vi "Get_WT_Speed.vi"(2 "Time (s)":dbl[](array[numeric]) format="%.4f", 3 "Av Sampling Rate":dbl, 4 "Opto Trace":dbl[](array[numeric]) format="%.2f") -> (0 "Time per Cycle":dbl[](array[numeric]), 1 "Start Cycle Time":dbl[](array[numeric]))   [LabVIEW 2021]
uses:
  <vilib>/Analysis/6fits.llb/Curve Fitting Criteria.ctl
  <vilib>/Analysis/baseanly.llb/Mean (DBL).vi
  <vilib>/Analysis/NI_AALBase.lvlib
  <vilib>/Analysis/NI_AALPro.lvlib
panel:
  out "Samples per cycle 1st":i32[](graph)
  out "Time (s) per cycle":dbl[](graph)
  out "Threshold value":dbl
  out "1/60 of cycle":i32
  out "Average samples per cycle":dbl format="%0.2f"
  out "No Of Cycles":i32
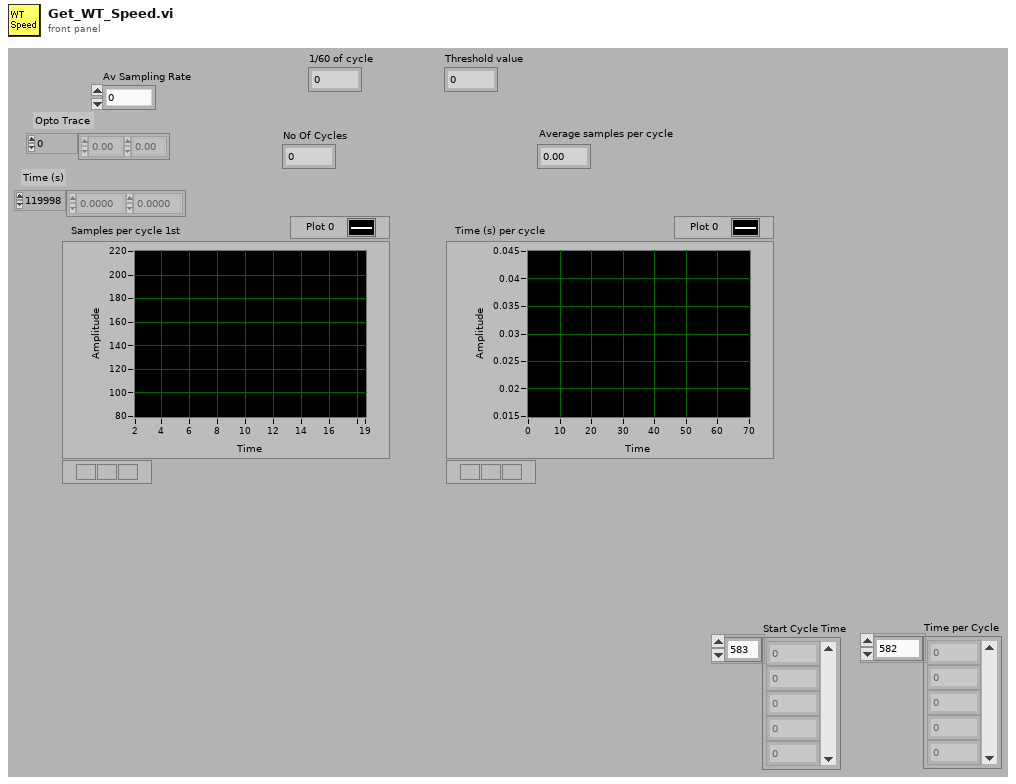
[diagram p1: front panel]
types:
  T1 = typedef "NI_AALPro.lvlib/Curve Fitting Criteria.ctl" = u16
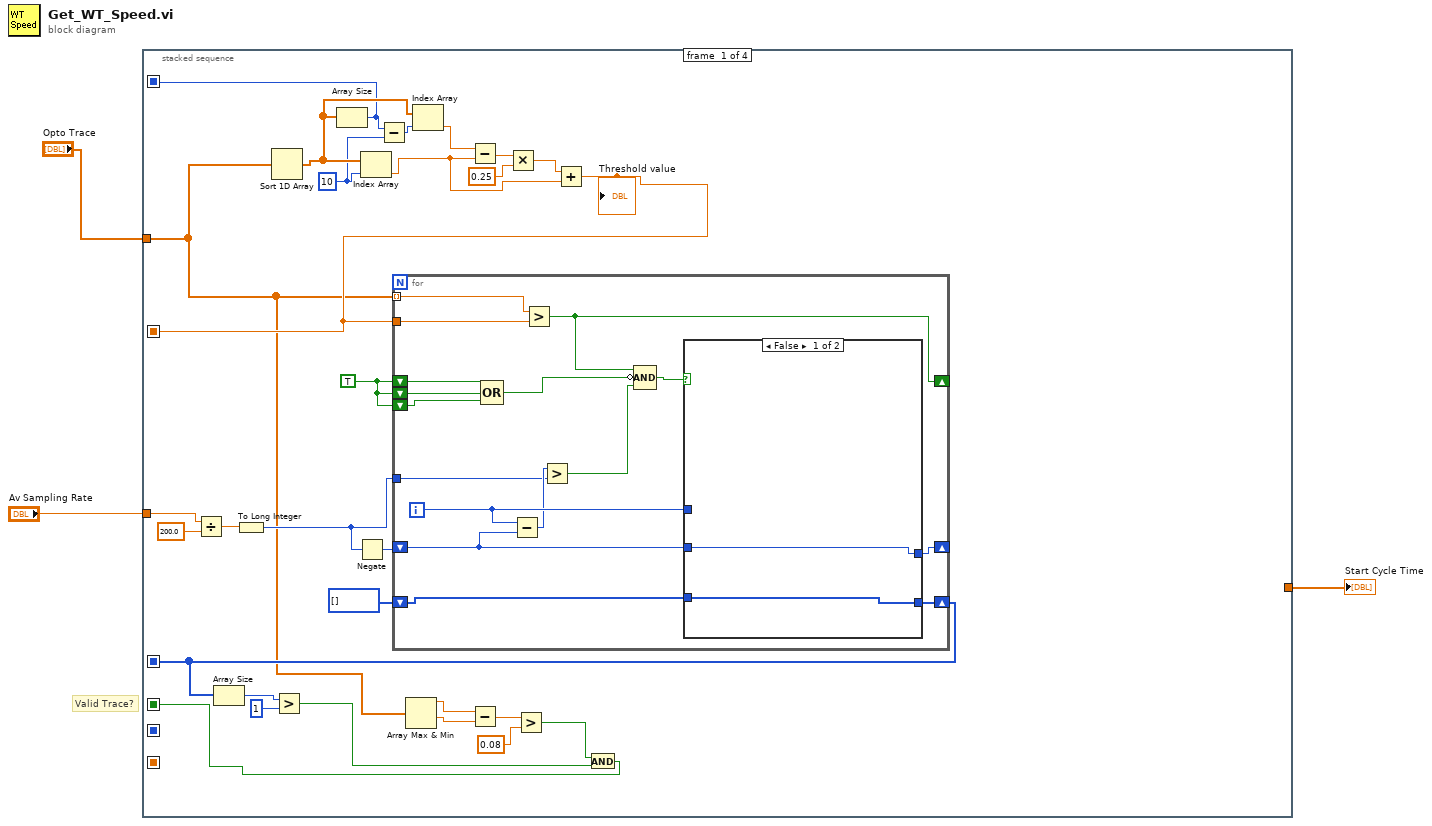
[diagram p0: block diagram]
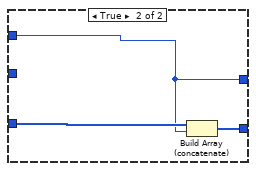
[diagram p2: hidden frame]
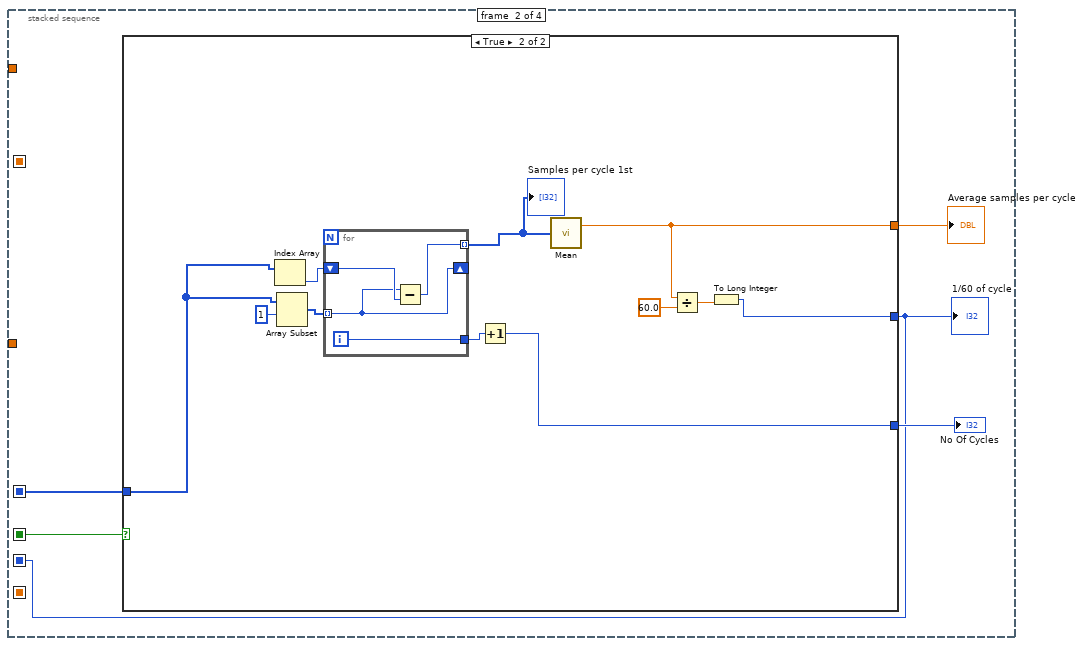
[diagram p3: hidden frame]
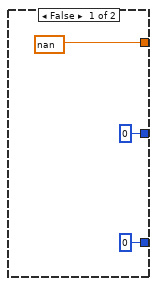
[diagram p4: hidden frame]
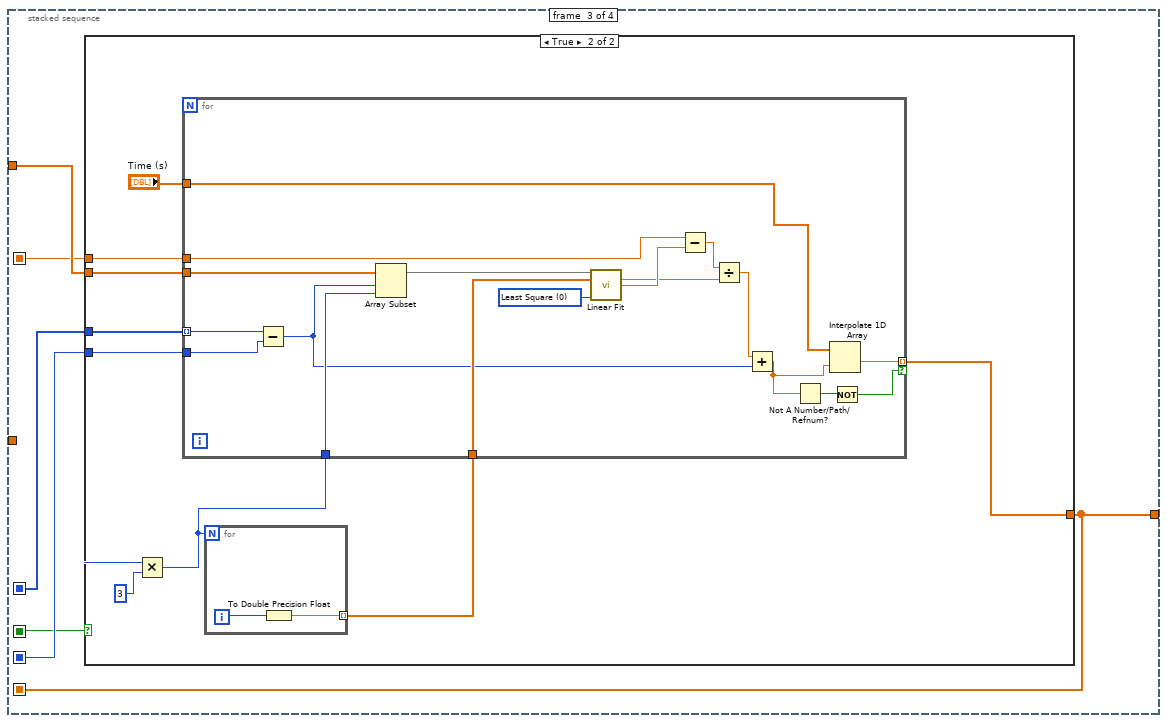
[diagram p5: hidden frame]
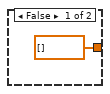
[diagram p6: hidden frame]
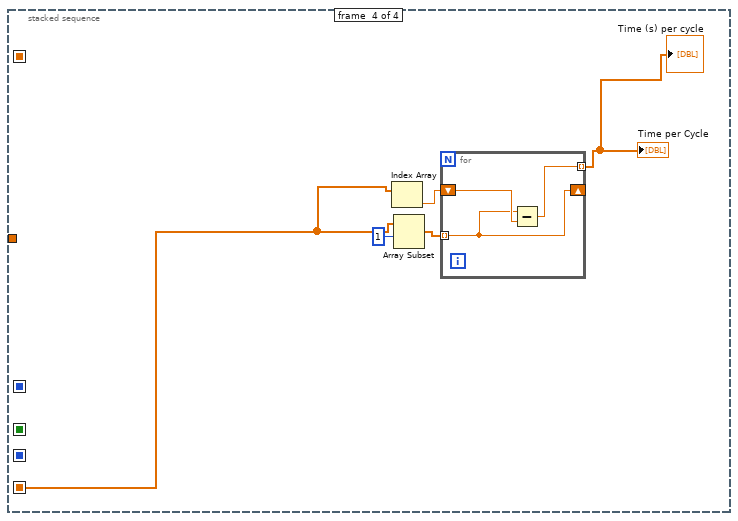
[diagram p7: hidden frame]
diagram:
  # "Valid Trace?"
  n1 = stacked-sequence {
    seq-local: [w14 _ _ _] -> [_ w55 w81 _]
    seq-local: [w20 _ _ _] -> [_ _ _ _]
    seq-local: [_ w56 _ _] -> [_ _ w80 _]
    seq-local: [w19 _ _ _] -> [_ _ w78 _]
    seq-local: [_ _ w77 _] -> [_ _ _ w113]
    seq-local: [w4 _ _ _] -> [_ w53 w76 _]
    tunnel: [_ _ w77 _] -> w3
    tunnel: "Av Sampling Rate" -> [w18 _ _ _]
    tunnel: "Opto Trace" -> [w11 _ w79 _]
    frame #0 {
      w22 = TRUE
      w29 = 10 ("index")
      n2 = Divide(x=w18, y=200.0) -> (x/y=w16:dbl)
      n3 = To Long Integer(number=w16) -> (32bit integer=w15:i32)
      n4 = Sort 1D Array(array=w11) -> (sorted array=w31:dbl[])
      n5 = Array Size(array=w31) -> (size(s)=w20:i32)
      n6 = Negate(x=w15) -> (-x=w21:i32)
      n7 = Index Array(array=w31, index=w29) -> (element=w23:dbl)
      n8 = Subtract(x=w20, y=w29) -> (x-y=w30:i32)
      n9 = Array Max & Min(array=w11) -> (max value=w10:dbl, min value=w9:dbl)  [unwired: 2 out]
      n10 = Index Array(array=w31, index=w30) -> (element=w27:dbl)
      n11 = Subtract(x=w27, y=w23) -> (x-y=w26:dbl)
      n12 = Subtract(x=w10, y=w9) -> (x-y=w8:dbl)
      n13 = Multiply(x=w26, y=0.25) -> (x*y=w24:dbl)
      n14 = Greater?(x=w8, y=0.08) -> (0:w6:bool)
      n15 = Add(x=w24, y=w23) -> (x+y=w19:dbl)
      "Threshold value" <- w19
      n16 = for {
        shift-right: [w38] -> _
        shift-left: w22 -> [w42]
        tunnel: w11 -> [w47] mode=indexing
        tunnel: w19 -> [w46]
        shift-right: [w43] -> w14
        shift-left: i32[] [] -> [w44]
        shift-left: w22 -> [w41]
        shift-left: w22 -> [w40]
        shift-right: [w37] -> _
        shift-left: w21 -> [w35]
        tunnel: w15 -> [w33]
        i -> [w36]
        n17 = Compound Arithmetic op=OR(w42, w41, w40) -> (w39:bool)
        n18 = Subtract(x=w36, y=w35) -> (x-y=w34:i32)
        n19 = Greater?(x=w47, y=w46) -> (0:w38:bool)
        n20 = Greater?(x=w34, y=w33) -> (0:w32:bool)
        n21 = Compound Arithmetic op=AND(w38, invert w39, w32) -> (w45:bool)
        n22 = case shown="False" w45 {
          tunnel: w36 -> [_ w50]
          tunnel: w44 -> [w49 w52]
          tunnel: [w49 w51] -> w43
          tunnel: [w48 w50] -> w37
          tunnel: w35 -> [w48 _]
          frame False {
          }
          frame True {
            n23 = Build Array (concatenate)(w52, w50) -> (w51:i32[])
          }
        }
      }
      n24 = Array Size(array=w14) -> (size(s)=w13:i32)
      n25 = Greater?(x=w13, y=1) -> (0:w5:bool)
      n26 = And(x=w6, y=w5) -> (x .and. y?=w4:bool)
    }
    frame #1 {
      n27 = case shown="True" w53 {
        tunnel: [0 w67] -> w57
        tunnel: [0 w64] -> w56
        tunnel: w55 -> [_ w63]
        tunnel: [nan w62] -> w54
        frame False {
        }
        frame True {
          n28 = Index Array(array=w63) -> (element=w69:i32)  [unwired: 1 in]
          n29 = Array Subset(array=w63, index=1) -> (w70:i32[])  [unwired: 1 in]
          n30 = for {
            shift-right: [w74] -> _
            shift-left: w69 -> [w75]
            tunnel: w70 -> [w74] mode=indexing
            tunnel: [w73] -> w61 mode=indexing
            tunnel: [w72] -> w71
            i -> [w72]
            n31 = Subtract(x=w74, y=w75) -> (x-y=w73:i32)
          }
          "Samples per cycle 1st" <- w61
          n32 = Increment(x=w71) -> (x+1=w67:i32)
          n33 = call-poly <vilib>:"Mean.vi"("X"=w61) -> ("mean"=w62:dbl)  [unwired: 1 out]
          n34 = Divide(x=w62, y=60.0) -> (x/y=w65:dbl)
          n35 = To Long Integer(number=w65) -> (32bit integer=w64:i32)
        }
      }
      "No Of Cycles" <- w57
      "Average samples per cycle" <- w54
      "1/60 of cycle" <- w56
    }
    frame #2 {
      n36 = case shown="True" w76 {
        tunnel: w81 -> [_ w91]
        tunnel: w80 -> [_ w90]
        tunnel: w79 -> [_ w87]
        tunnel: w78 -> [_ w85]
        tunnel: [dbl[] [] w84] -> w77
        frame False {
        }
        frame True {
          n37 = Multiply(x=w90, y=3) -> (x*y=w86:i32)
          n38 = for {
            N: w86 -> [_]
            tunnel: [w92] -> w88 mode=indexing
            i -> [w93]
            n39 = To Double Precision Float(number=w93) -> (double precision float=w92:dbl)
          }
          n40 = for {
            tunnel: w91 -> [w111] mode=indexing
            tunnel: w90 -> [w110]
            tunnel: w88 -> [w109]
            tunnel: w87 -> [w108]
            tunnel: w86 -> [w107]
            tunnel: w85 -> [w104]
            tunnel: [w97] -> w84 mode=indexing if=w94
            tunnel: "Time (s)" -> [w98]
            w105 = T1 0 items=["Least Square", "Least Absolute Residual", "Bisquare"] ("method")
            n41 = Subtract(x=w111, y=w110) -> (x-y=w99:i32)
            n42 = Array Subset(array=w108, index=w99, length=w107) -> (w106:dbl[])
            n43 = call <vilib>:"Linear Fit.vi"("Y"=w106, "X"=w109, "method"=w105) -> ("slope"=w101:dbl, "intercept"=w103:dbl)  [unwired: 8 in, 3 out]
            n44 = Subtract(x=w104, y=w103) -> (x-y=w102:dbl)
            n45 = Divide(x=w102, y=w101) -> (x/y=w100:dbl)
            n46 = Add(x=w100, y=w99) -> (x+y=w96:dbl)
            n47 = Not A Number/Path/Refnum?(number/path/refnum=w96) -> (NaN/Path/Refnum?=w95:bool)
            n48 = Interpolate 1D Array(1:w96, 2:w98) -> (0:w97:dbl)
            n49 = Not(x=w95) -> (.not. x?=w94:bool)
          }
        }
      }
    }
    frame #3 {
      n50 = Index Array(array=w113) -> (element=w115:dbl)  [unwired: 1 in]
      n51 = Array Subset(array=w113, index=1) -> (w116:dbl[])  [unwired: 1 in]
      n52 = for {
        shift-right: [w118] -> _
        shift-left: w115 -> [w119]
        tunnel: w116 -> [w118] mode=indexing
        tunnel: [w117] -> w112 mode=indexing
        n53 = Subtract(x=w118, y=w119) -> (x-y=w117:dbl)
      }
      "Time per Cycle" <- w112
      "Time (s) per cycle" <- w112
    }
  }
  "Start Cycle Time" <- w3
